vi "Grpc LabVIEW Proto Generator.vi"(0 "Proto File Path":path[](array[path]), 1 "Generated Library Name":string, 2 "Library Suffix":string caption="Generated Library Suffix (\"_server\" / \"_client\" by default, if empty)", 3 "Generate":enum16{"gRPC Server", "gRPC Client", "Both"}(ring), 5 "Import Paths":path[](array[path]), 7 "Prototype Library":path, 9 "Target Project":path, 11 "error in (no error)":errorcluster) -> (15 "error out":errorcluster)   [LabVIEW 2020]
panel:
  # "This is a wrapper to the grpc-labview generator utility, which allows for programmatic execution via VIServer.\n\nLast update was against v0.5.2.2 of the utility."
  # "Ignored for servers as of v0.5.2.2"
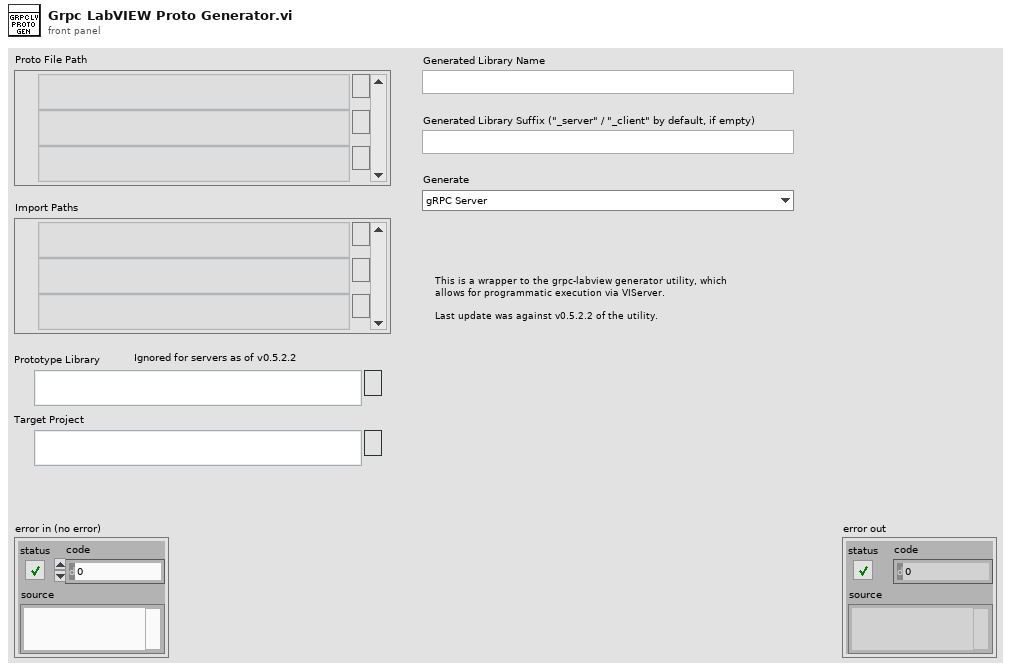
[diagram p1: front panel]
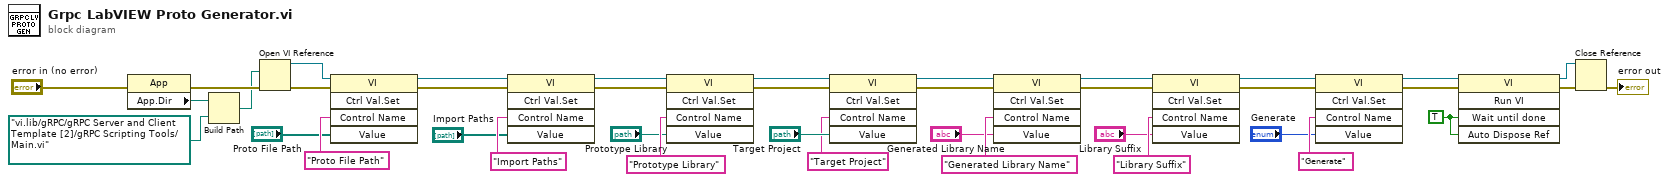
[diagram p0: block diagram]
diagram:
  w4 = TRUE ("Wait Until Done")
  n1 = property class="App"(error in="error in (no error)") -> (error out=w36:errorcluster, "App.Dir"=w39:path)  [unwired: 1 in, 1 out]
  n2 = Build Path(base path=w39, name or relative path=path "vi.lib/gRPC/gRPC Server and Client Template [2]/gRPC Scripting Tools/Main.vi" ("Target Project")) -> (appended path=w35:path)
  n3 = Open VI Reference(vi path=w35, error in (no error)=w36) -> (vi reference=w33:refnum<vi>, error out=w34:errorcluster)  [unwired: 4 in]
  n4 = invoke class="VI" method="Ctrl Val.Set"(reference=w33, error in=w34, "Control Name"="Proto File Path", "Value"="Proto File Path") -> (reference out=w28:refnum<vi>, error out=w29:errorcluster)  [unwired: 1 in, 3 out]
  n5 = invoke class="VI" method="Ctrl Val.Set"(reference=w28, error in=w29, "Control Name"="Import Paths", "Value"="Import Paths") -> (reference out=w23:refnum<vi>, error out=w24:errorcluster)  [unwired: 1 in, 3 out]
  n6 = invoke class="VI" method="Ctrl Val.Set"(reference=w23, error in=w24, "Control Name"="Prototype Library", "Value"="Prototype Library") -> (reference out=w20:refnum<vi>, error out=w21:errorcluster)  [unwired: 1 in, 3 out]
  n7 = invoke class="VI" method="Ctrl Val.Set"(reference=w20, error in=w21, "Control Name"="Target Project", "Value"="Target Project") -> (reference out=w13:refnum<vi>, error out=w14:errorcluster)  [unwired: 1 in, 3 out]
  n8 = invoke class="VI" method="Ctrl Val.Set"(reference=w13, error in=w14, "Control Name"="Generated Library Name", "Value"="Generated Library Name") -> (reference out=w16:refnum<vi>, error out=w15:errorcluster)  [unwired: 1 in, 3 out]
  n9 = invoke class="VI" method="Ctrl Val.Set"(reference=w16, error in=w15, "Control Name"="Library Suffix", "Value"="Library Suffix") -> (reference out=w18:refnum<vi>, error out=w17:errorcluster)  [unwired: 1 in, 3 out]
  n10 = invoke class="VI" method="Ctrl Val.Set"(reference=w18, error in=w17, "Control Name"="Generate", "Value"="Generate") -> (reference out=w6:refnum<vi>, error out=w5:errorcluster)  [unwired: 1 in, 3 out]
  n11 = invoke class="VI" method="Run VI"(reference=w6, error in=w5, "Wait until done"=w4, "Auto Dispose Ref"=w4) -> (reference out=w3:refnum<vi>, error out=w2:errorcluster)  [unwired: 1 in, 3 out]
  n12 = Close Reference(reference=w3, error in (no error)=w2) -> (error out=→"error out":errorcluster)
